vi "Test Test Run Result not Returned by Test Suite.vi"(8 "error in (no error)":errorcluster, 11 "LUnit Test Suite Tests In":refnum<class "LUnit Test Suite Tests.lvclass">) -> (0 "error out":errorcluster, 3 "LUnit Test Suite Tests Out":refnum<class "LUnit Test Suite Tests.lvclass">)   [LabVIEW 2020, in "LUnit Test Suite Tests.lvclass"]
uses:
  LUnit Test Suite Tests.lvclass
  LUnit Test Suite Tests.lvclass/LUnit Test Suite Tests.ctl
  b74e4934-f044-4222-b3dd-fc90e6c1bd4f.vi
  source/LUnit Test Suite.lvclass
  Test Doubles/Test Case Test Double Child/Light Test Case Double.lvclass
  source/Core/Result/Type.ctl
  source/Core/Result/Result.lvlib
  C:/git/astemes-lunit/source/Core/Runnable/Runnable.lvclass
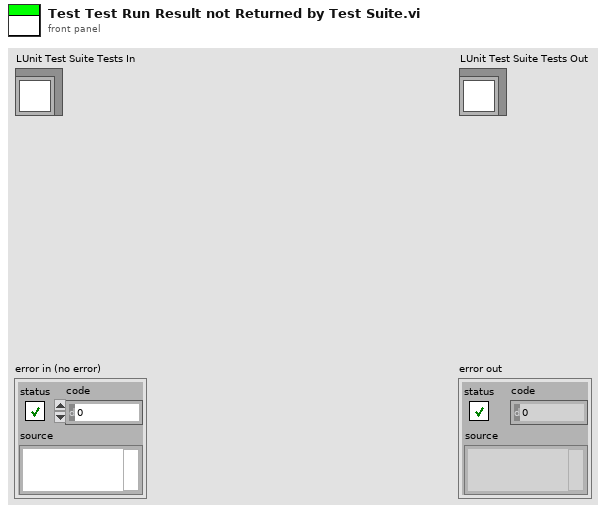
[diagram p1: front panel]
types:
  T1 = typedef "Result.lvlib/Result.ctl" = cluster{"Name":string, "Description":string, "Status":T2, "Result Type":T3, "Execution Time":dbl, "Data":cluster{"Expected":variant, "Actual":variant, "Delta":variant}}
  T2 = typedef "Result.lvlib/Status.ctl" = enum16{"", "Passed", "Failed", "Error", "Skipped", "Setup Error", "Broken", "Teardown Error"}
  T3 = typedef "Result.lvlib/Type.ctl" = enum16{"Test Case", "Test Suite", "Test Run", "Pass", "Fail", "Skip", "Pass if", "Fail if", "Pass if Error", "Fail if Error", "Pass if Equal", "Fail if Equal"}
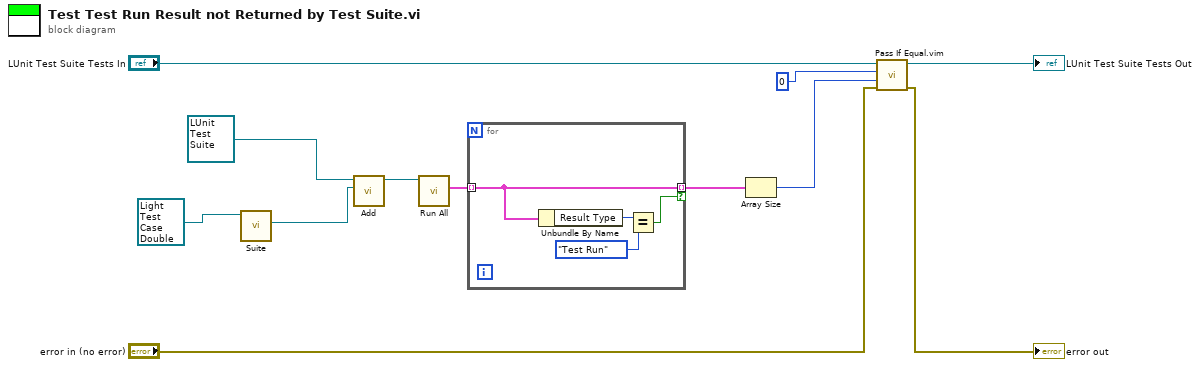
[diagram p0: block diagram]
diagram:
  n1 = call-dynamic "Suite.vi"("LUnit Test Case In"=refnum<class "Light Test Case Double.lvclass"> refnum ("Light Test Case Double.lvclass")) -> ("LUnit Test Suite Out"=w1:refnum<class "LUnit Test Suite.lvclass">)  [unwired: 8 in, 2 out]
  n2 = call "Add.vi"("Runnable"=w1, "LUnit Test Suite In"=refnum<class "LUnit Test Suite.lvclass"> refnum ("Run in")) -> ("LUnit Test Suite Out"=w6:refnum<class "LUnit Test Suite.lvclass">)  [unwired: 8 in, 1 out]
  n3 = call "Run All.vi"("Runnable In"=w6) -> ("Results"=w4:T1[])  [unwired: 9 in, 1 out]
  n4 = for {
    tunnel: w4 -> [w14] mode=indexing
    tunnel: [w14] -> w3 mode=indexing if=w13
    n5 = Unbundle By Name(w14) -> ("Result Type"=w16:T3)
    n6 = Equal?(x=w16, y=Type."Test Run") -> (x = y?=w13:bool)
  }
  n7 = Array Size(array=w3) -> (size(s)=w8:i32)
  n8 = call "Pass If Equal.vim"("error in (no error)"="error in (no error)", "Actual"=w8, "Expected"=0 ("size(s)"), "LUnit Test Case In"="LUnit Test Suite Tests In") -> ("error out"=→"error out":errorcluster, "LUnit Test Case Out"=→"LUnit Test Suite Tests Out":refnum<class "LUnit Test Suite Tests.lvclass">)  [unwired: 6 in]
